vi "frequency_to_flow_volume.vi"(9 "mlL/pulse":dbl, 10 "Pulse Count":dbl, 11 "Pulse Frequency [Hz]":dbl) -> (2 "Volume [L]":dbl, 3 "Flow [L/min]":dbl)   [LabVIEW 2025, in "LabJackEKG.lvlib"]
uses:
  LabJackEKG.lvlib
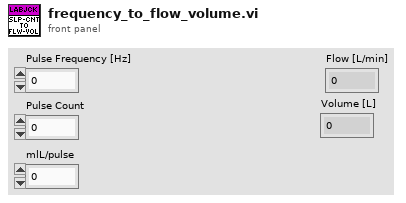
[diagram p1: front panel]
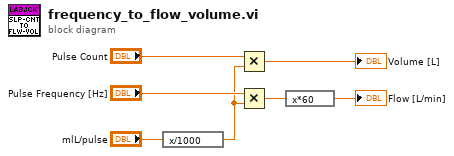
[diagram p0: block diagram]
diagram:
  n1 = expression code="x/1000"("mlL/pulse") -> (w1:dbl)
  n2 = Multiply(x="Pulse Count", y=w1) -> (x*y=→"Volume [L]":dbl)
  n3 = Multiply(x="Pulse Frequency [Hz]", y=w1) -> (x*y=w6:dbl)
  n4 = expression code="x*60"(w6) -> (→"Flow [L/min]":dbl)
